vi "Modbus Init.vi"(8 "error in (no error)":errorcluster, 10 "Modbus Port (Port, Baudrate)":T1={"COM Port"="COM3", "Baud Rate"=9600}) -> (0 "error out":errorcluster, 3 "VISA resource out":refnum<visa-resource-name>)   [LabVIEW 2024, in "Voegtlin_NI_SMART_Modbus_Drivers.lvlib"]
doc: "Baut eine Modbus-Verbingung ueber den angegebene COM-Port auf."
uses:
  Voegtlin_NI_SMART_Modbus_Drivers.lvlib
  Port.ctl
  Low Level Driver/Enums/Modbus Comm.ctl
panel:
  # "Output Data"
  # "Input Data"
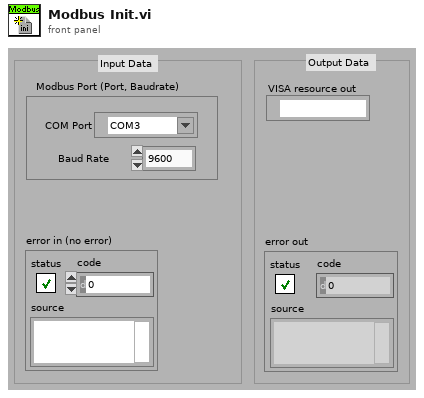
[diagram p1: front panel]
types:
  T1 = typedef "Voegtlin_NI_SMART_Modbus_Drivers.lvlib/Port.ctl" = cluster{"COM Port":refnum<visa-resource-name>, "Baud Rate":u32}
  T2 = typedef "Voegtlin_NI_SMART_Modbus_Drivers.lvlib/Modbus Comm.ctl" = enum16{"Init", "Read", "Write", "Exit"}
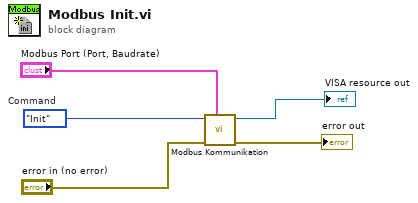
[diagram p0: block diagram]
diagram:
  w2 = Modbus_Comm."Init"  # Command
  n1 = call "Modbus Kommunikation.vi"("Modbus Port (Port,  Baudrate)"="Modbus Port (Port, Baudrate)", "error in (no error)"="error in (no error)", "Command"=w2) -> ("error out"=→"error out":errorcluster, "VISA resource out"=→"VISA resource out":refnum<visa-resource-name>)  [unwired: 6 in, 1 out]
